vi "init_photosensor.vi"(6 "error in":errorcluster, 7 "Physical Channel":tag="Dev1/ai0", 8 "Number of Samples":i32=100, 9 "Sample Rate":dbl=1000.0, 10 "Min Voltage":dbl=-5.0, 11 "Max Voltage":dbl=5.0) -> (3 "task out":refnum<k21>, 4 "error out":errorcluster)   [LabVIEW 2018]
doc: "This VI initializes a DAQ channel settings"
uses:
  SupportVIs/DAQmx Create Channel (AI-Voltage-Basic).vi
  SupportVIs/DAQmx Timing (Sample Clock).vi
  C:/Program Files/National Instruments/LabVIEW 2018/resource/objmgr/daqmx.rc
panel:
  in  "Sample Clock Source":tag="OnboardClock"
  in  "Terminal Configuration":i32(ring)=-1 items=["default"=-1, "RSE"=10083, "NRSE"=10078, "Differential"=10106, "Pseudodifferential"=12529]
  out "Actual Sample Rate":dbl=1000.0 format="%0.2f"
  # "Channel Settings"
  # "Timing Settings"
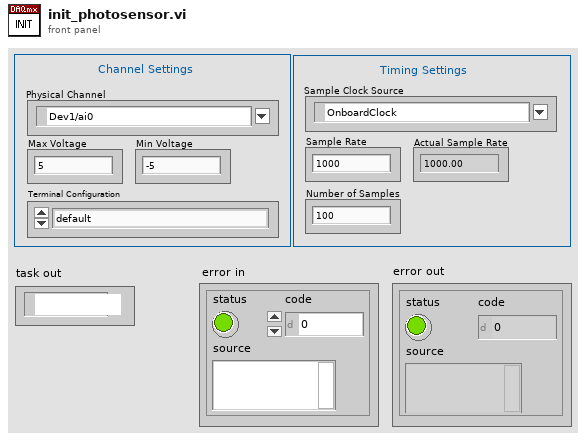
[diagram p1: front panel]
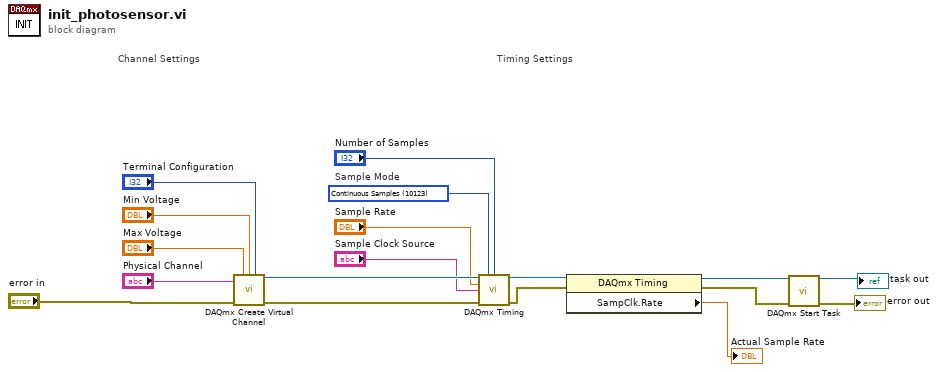
[diagram p0: block diagram]
diagram:
  w16 = 10123 items=["Finite Samples"=10178, "Continuous Samples"=10123, "Hardware Timed Single Point"=12522]  # Sample Mode
  # "Timing Settings"
  # "Channel Settings"
  n1 = call-poly "DAQmx Create Virtual Channel.vi"("maximum value"="Max Voltage", "minimum value"="Min Voltage", "input terminal configuration"="Terminal Configuration", "physical channels"="Physical Channel", "error in"="error in") -> ("task out"=w14:refnum<k21>, "error out"=w15:errorcluster)  [unwired: 9 in]
  n2 = call-poly "DAQmx Timing.vi"("task/channels in"=w14, "sample mode"=w16, "samples per channel"="Number of Samples", "rate"="Sample Rate", "source"="Sample Clock Source", "error in"=w15) -> ("task out"=w18:refnum<k21>, "error out"=w17:errorcluster)  [unwired: 8 in]
  n3 = property class="DAQmx Timing"(reference=w18, error in=w17) -> (reference out=w5:refnum<k21>, error out=w4:errorcluster, "SampClk.Rate"=→"Actual Sample Rate":dbl)
  n4 = call "DAQmx Start Task.vi"("task/channels in"=w5, "error in"=w4) -> ("task out"=→"task out":refnum<k21>, "error out"=→"error out":errorcluster)  [unwired: 12 in]
